vi "FRCts20_EspEngine_Team.vi"(8 "error in (no error)":errorcluster, 10 "Team":T1, 11 "httpRequestID":u32) -> (0 "error out":errorcluster, 3 "httpRequestID out":u32)   [LabVIEW 2014, in "FRCts20_EspEngine.lvlib"]
uses:
  FRCts20_EspEngine.lvlib
  TypeDefs/FRCts20_EspEngine_Team.ctl
  Web Methods/source/VI Source/Web Method Public Interface/FRCts20_WebMethods_ctl_singleTeam.ctl
  Web Methods/source/VI Source/Web Method Public Interface/FRCts20_WebMethods_ctl_teamIdentifier.ctl
  Backend/source/VI Source/FRCts20_Backend_API/FRCts20_Backend_API_SW.ctl
  Web Methods/source/VI Source/Web Method Public Interface/FRCts20_WebMethods_ctl_request.ctl
  Backend/source/VI Source/FRCts20_Backend_API/FRCts20_Backend_API_Status.ctl
  <vilib>/wsapi/subVIs/Set Integer ESP Variable.vi
  <vilib>/wsapi/subVIs/Set String ESP Variable.vi
  FRCts20_EspEngine_FormatArrayOfKeysInts.vi
  FRCts20_EspEngine_FormatArrayOfKeysStrings.vi
  <vilib>/wsapi/NI_WebServices.lvlib
  Web Methods/source/VI Source/FRCts20_WebMethods.lvlib
  Backend/source/VI Source/FRCts20_Backend_API/FRCts20_Backend_API.lvlib
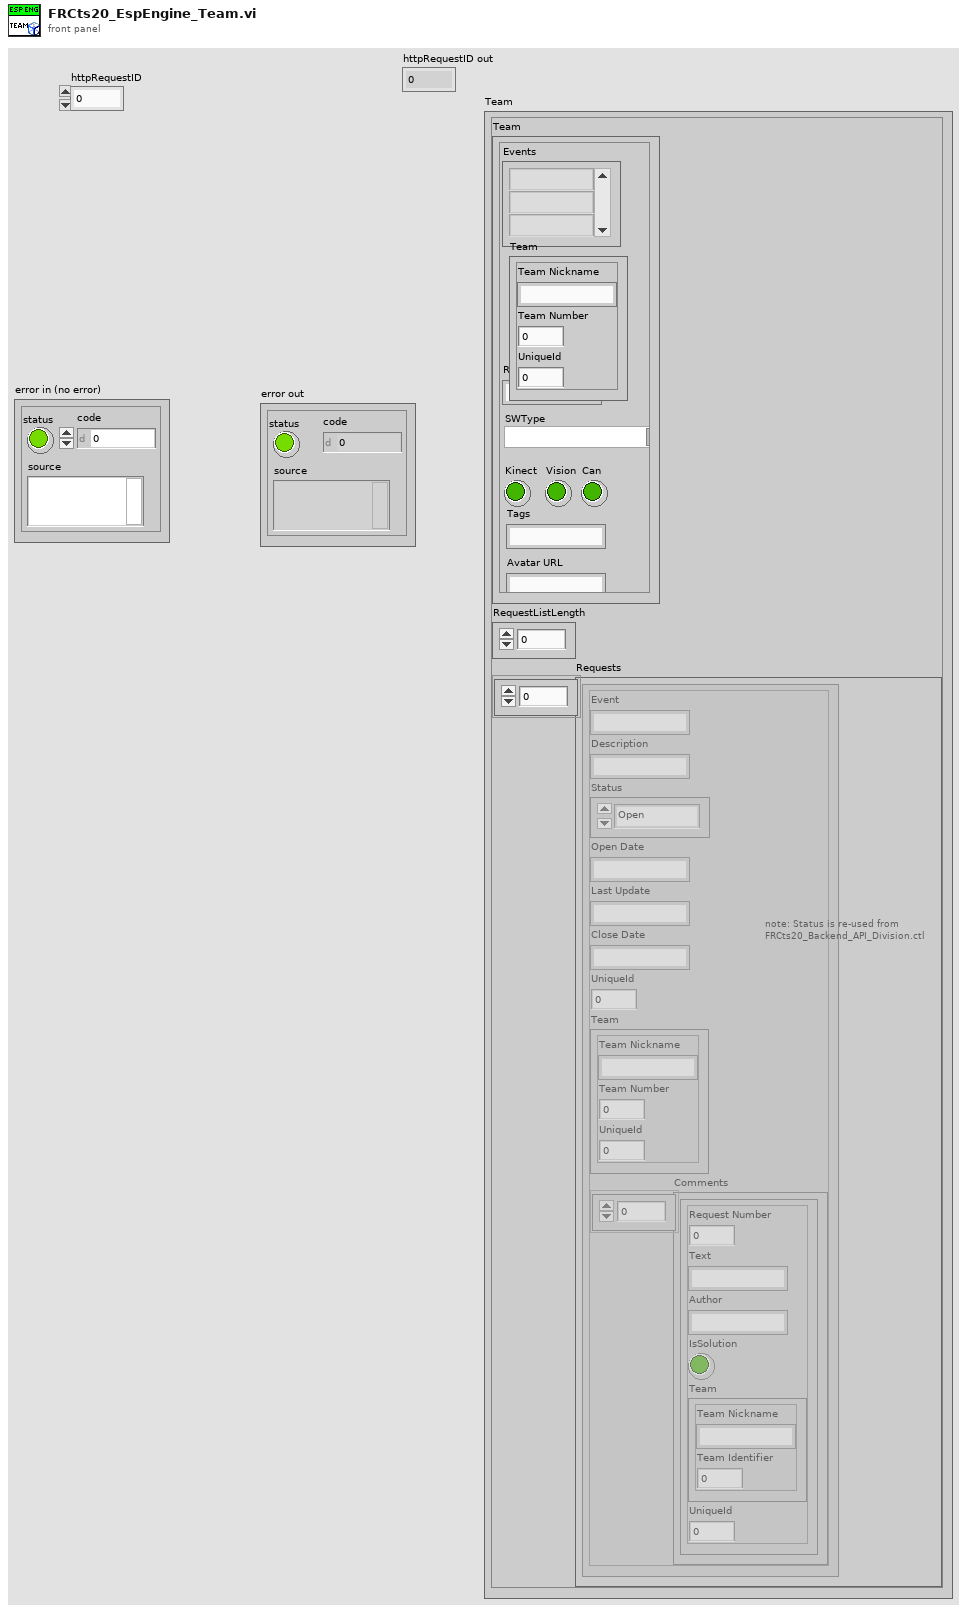
[diagram p1: front panel]
types:
  T1 = typedef "FRCts20_EspEngine.lvlib/FRCts20_EspEngine_Team.ctl" = cluster{"Team":T2, "RequestListLength":i16, "Requests":T5[]}
  T2 = typedef "FRCts20_WebMethods.lvlib/FRCts20_WebMethods_ctl_singleTeam.ctl" = cluster{"Events":string[], "Robot Name":string, "Kinect":bool, "Vision":bool, "Can":bool, "Tags":string, "Avatar URL":string, "Team":T3, "SWType":T4}
  T3 = typedef "FRCts20_WebMethods.lvlib/FRCts20_WebMethods_ctl_teamIdentifier.ctl" = cluster{"Team Nickname":string, "Team Number ":u32, "UniqueId":u32}
  T4 = typedef "FRCts20_Backend_Engine.lvlib/FRCts20_Backend_API.lvlib/FRCts20_Backend_API_SW.ctl" = string
  T5 = typedef "FRCts20_WebMethods.lvlib/FRCts20_WebMethods_ctl_request.ctl" = cluster{"Event":string, "Description":string, "Status":T6, "Open Date":string, "Last Update":string, "Close Date":string, "UniqueId":i32, "Team":cluster{"Team Nickname":string, "Team Number ":i32, "UniqueId":i32}, "Comments":cluster{"Request Number":dbl, "Text":string, "Author":string, "IsSolution":bool, "Team":cluster{"Team Nickname":string, "Team Identifier ":dbl}, "UniqueId":i32}[]}
  T6 = typedef "FRCts20_Backend_Engine.lvlib/FRCts20_Backend_API.lvlib/FRCts20_Backend_API_Status.ctl" = enum16{"Open", "In Work", "Closed"}
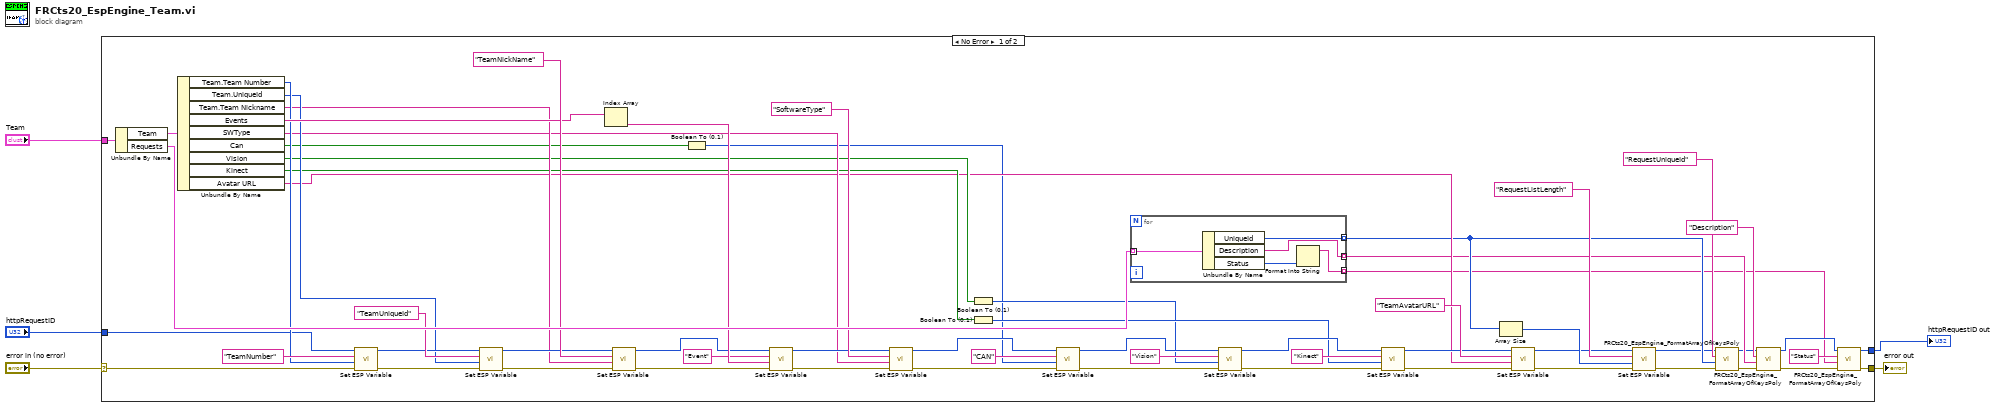
[diagram p0: block diagram]
diagram:
  n1 = case shown="No Error" "error in (no error)" {
    selector: "error in (no error)" -> [w11 w72]
    tunnel: [w12 w72] -> w5
    tunnel: "Team" -> [w66 _]
    tunnel: "httpRequestID" -> [w43 _]
    tunnel: [w9 _] -> w1
    frame No Error {
      n2 = Unbundle By Name(w66) -> ("Team"=w65:T2, "Requests"=w64:T5[])
      n3 = Unbundle By Name(w65) -> ("Team.Team Number"=w44:u32, "Team.UniqueId"=w34:u32, "Team.Team Nickname"=w33:string, "Events"=w52:string[], "SWType"=w32:T4, "Can"=w31:bool, "Vision"=w30:bool, "Kinect"=w29:bool, "Avatar URL"=w28:string)
      n4 = call-poly <vilib>:"Set ESP Variable.vi"("error in (no error)"=w11, "value"=w44, "key"="TeamNumber", "httpRequestID"=w43) -> ("error out"=w63:errorcluster, "httpRequestID out"=w42:u32)  [unwired: 6 in]
      n5 = call-poly <vilib>:"Set ESP Variable.vi"("error in (no error)"=w63, "value"=w34, "key"="TeamUniqueId", "httpRequestID"=w42) -> ("error out"=w62:errorcluster, "httpRequestID out"=w41:u32)  [unwired: 6 in]
      n6 = Index Array(array=w52) -> (element=w51:string)  [unwired: 1 in]
      n7 = call-poly <vilib>:"Set ESP Variable.vi"("error in (no error)"=w62, "value"=w33, "key"="TeamNickName", "httpRequestID"=w41) -> ("error out"=w60:errorcluster, "httpRequestID out"=w40:u32)  [unwired: 6 in]
      n8 = Boolean To (0,1)(Boolean=w31) -> (0, 1=w6:i16)
      n9 = call-poly <vilib>:"Set ESP Variable.vi"("error in (no error)"=w60, "value"=w51, "key"="Event", "httpRequestID"=w40) -> ("error out"=w61:errorcluster, "httpRequestID out"=w39:u32)  [unwired: 6 in]
      n10 = call-poly <vilib>:"Set ESP Variable.vi"("error in (no error)"=w61, "value"=w32, "key"="SoftwareType", "httpRequestID"=w39) -> ("error out"=w59:errorcluster, "httpRequestID out"=w38:u32)  [unwired: 6 in]
      n11 = Boolean To (0,1)(Boolean=w30) -> (0, 1=w7:i16)
      n12 = Boolean To (0,1)(Boolean=w29) -> (0, 1=w8:i16)
      n13 = call-poly <vilib>:"Set ESP Variable.vi"("error in (no error)"=w59, "value"=w6, "key"="CAN", "httpRequestID"=w38) -> ("error out"=w58:errorcluster, "httpRequestID out"=w37:u32)  [unwired: 6 in]
      n14 = for {
        tunnel: w64 -> [w71] mode=indexing
        tunnel: [w70] -> w24 mode=indexing
        tunnel: [w69] -> w20 mode=indexing
        tunnel: [w67] -> w14 mode=indexing
        n15 = Unbundle By Name(w71) -> ("UniqueId"=w70:i32, "Description"=w69:string, "Status"=w68:T6)
        n16 = Format Into String(w68) -> (resulting string=w67:string)  [unwired: 3 in, 1 out]
      }
      n17 = call-poly <vilib>:"Set ESP Variable.vi"("error in (no error)"=w58, "value"=w7, "key"="Vision", "httpRequestID"=w37) -> ("error out"=w57:errorcluster, "httpRequestID out"=w36:u32)  [unwired: 6 in]
      n18 = call-poly <vilib>:"Set ESP Variable.vi"("error in (no error)"=w57, "value"=w8, "key"="Kinect", "httpRequestID"=w36) -> ("error out"=w56:errorcluster, "httpRequestID out"=w35:u32)  [unwired: 6 in]
      n19 = Array Size(array=w24) -> (size(s)=w26:i32)
      n20 = call-poly <vilib>:"Set ESP Variable.vi"("error in (no error)"=w56, "value"=w28, "key"="TeamAvatarURL", "httpRequestID"=w35) -> ("error out"=w13:errorcluster, "httpRequestID out"=w10:u32)  [unwired: 6 in]
      n21 = call-poly <vilib>:"Set ESP Variable.vi"("error in (no error)"=w13, "value"=w26, "key"="RequestListLength", "httpRequestID"=w10) -> ("error out"=w23:errorcluster, "httpRequestID out"=w16:u32)  [unwired: 6 in]
      n22 = call-poly "FRCts20_EspEngine_FormatArrayOfKeysPoly.vi"("error IO"=w23, "Values"=w24, "KeyBaseName"="RequestUniqueId" ("key"), "httpRequestID"=w16) -> ("error IO"=w22:errorcluster, "httpRequestID out"=w17:u32)  [unwired: 6 in]
      n23 = call-poly "FRCts20_EspEngine_FormatArrayOfKeysPoly.vi"("error IO"=w22, "Values"=w20, "KeyBaseName"="Description" ("key"), "httpRequestID"=w17) -> ("error IO"=w19:errorcluster, "httpRequestID out"=w18:u32)  [unwired: 6 in]
      n24 = call-poly "FRCts20_EspEngine_FormatArrayOfKeysPoly.vi"("error IO"=w19, "Values"=w14, "KeyBaseName"="Status", "httpRequestID"=w18) -> ("error IO"=w12:errorcluster, "httpRequestID out"=w9:u32)  [unwired: 6 in]
    }
    frame Error {
    }
  }
  "httpRequestID out" <- w1
  "error out" <- w5
